vi "Fetch Acquired Data (4xI16).vi"(7 "Timeout (s)":i32=5, 8 "error out":errorcluster, 10 "Samples":i32=-1, 11 "FPGA Ref In":refnum<k20>) -> (0 "error out":errorcluster, 2 "Data":i16[](array[numeric]), 3 "FPGA RefOut":refnum<k20>, 4 "Elements Remaining":u32)   [LabVIEW 2012]
uses:
  <vilib>/Utility/error.llb/Error Cluster From Error Code.vi
  <vilib>/rvi/errors/niLvFpgaAdjustHostInterfaceError.vi
  <vilib>/rvi/interface/nirviMethod/nirviMethod.xnode
  <vilib>/rvi/errors/niLvFpgaMergeErrorWithErrorCode.vi
  <vilib>/FPGAPlugInAG/Dynamic/niLvFpga_ReadFifo_Dynamic.vi
panel:
  out "size(s)":i32
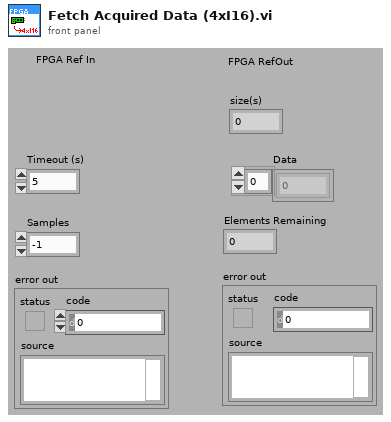
[diagram p1: front panel]
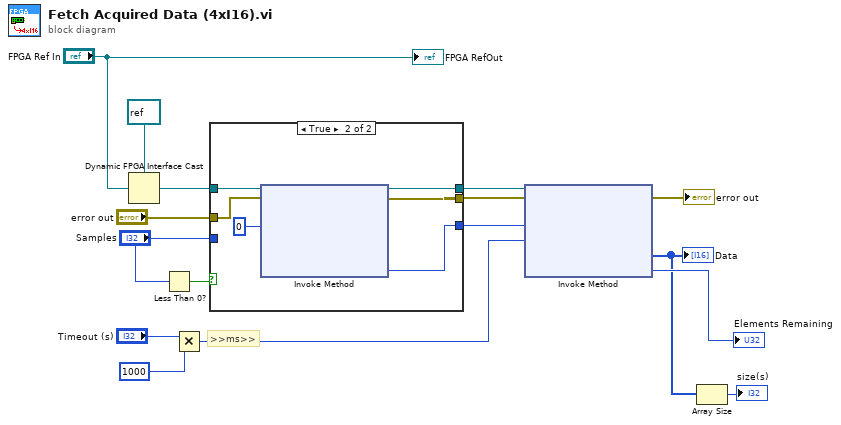
[diagram p0: block diagram]
diagram:
  # ">>ms>>"
  n1 = Dynamic FPGA Interface Cast(Session In=refnum<k20> refnum ("Type"), Type="FPGA Ref In") -> (Session Out=w7:refnum<k20>)
  n2 = Less Than 0?(x="Samples") -> (x < 0?=w14:bool)
  n3 = Multiply(x="Timeout (s)", y=1000) -> (x*y=w9:i32)
  n4 = case shown="True" w14 {
    tunnel: w7 -> [w18 w25]
    tunnel: "error out" -> [w19 w24]
    tunnel: [w18 w23] -> w12
    tunnel: [w19 w22] -> w11
    tunnel: [w17 w20] -> w5
    tunnel: "Samples" -> [w17 _]
    frame False {
    }
    frame True {
      n5 = xnode "Invoke Method"("FPGA VI Reference In"=w25, "error in"=w24, "Number of Elements"=u32 0) -> ("FPGA VI Reference Out"=w23:refnum<k20>, "error out"=w22:errorcluster, "Elements Remaining"=w20:u32)  [unwired: 1 in, 1 out]
    }
  }
  n6 = xnode "Invoke Method"("FPGA VI Reference In"=w12, "error in"=w11, "Number of Elements"=w5, "Timeout (ms)"=w9) -> ("error out"=→"error out":errorcluster, "Data"=w2:i16[], "Elements Remaining"=→"Elements Remaining":u32)  [unwired: 1 out]
  "Data" <- w2
  n7 = Array Size(array=w2) -> (size(s)=→"size(s)":i32)
  "FPGA RefOut" <- "FPGA Ref In"
